vi "LVOBJ to Variant.vi"(8 "error in (no error)":errorcluster, 9 "Variant Type":variant, 10 "JSON Path":string[](array[string]), 11 "Root":T1) -> (0 "error out":errorcluster, 2 "Key":string, 3 "Variant out":variant)   [LabVIEW 2019, in "labview_json.lvlib"]
uses:
  labview_json.lvlib
  Value.ctl
  Value Type.ctl
  <vilib>/Utility/Data Type/Type Definitions/Data Type.ctl
  <vilib>/Utility/error.llb/Error Cluster From Error Code.vi
  <vilib>/ErrorRing/Error Ring.xnode
  <vilib>/Utility/Data Type/NI_Data Type.lvlib
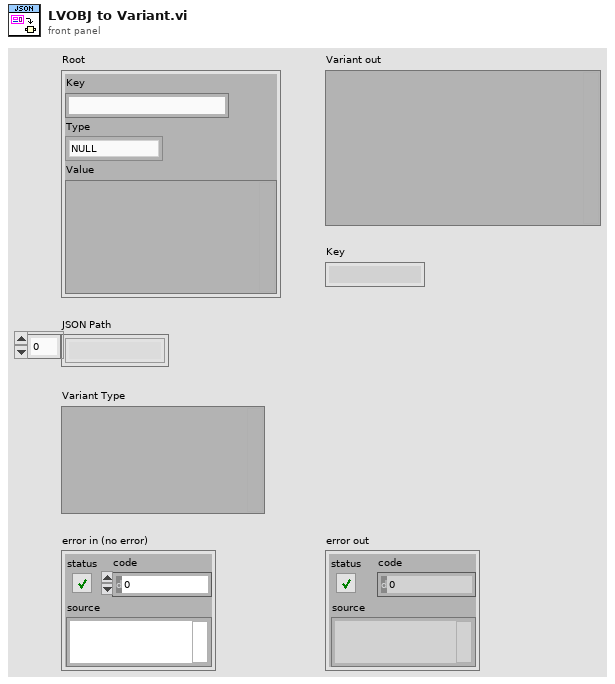
[diagram p1: front panel]
types:
  T1 = typedef "labview_json.lvlib/Value.ctl" = cluster{"Key":string, "Type":T2, "Value":variant}
  T2 = typedef "labview_json.lvlib/Value Type.ctl" = enum8{"NULL", "OBJECT", "ARRAY", "BOOL", "INT", "UINT", "FLOAT", "STRING"}
  T3 = typedef "NI_Data Type.lvlib/Data Type.ctl" = enum8{"Invalid Type", "Void", "I8", "I16", "I32", "I64", "U8", "U16", "U32", "U64", "Single Float", "Double Float", "Extended Float", "Single Complex", "Double Complex", "Extended Complex", "Enum U8", "Enum U16", "Enum U32", "Enum U64", "Single Float With Unit", "Double Float With Unit", "Extended Float With Unit", "Single Complex with Unit", "Double Complex with Unit", "Extended Complex with Unit", "Boolean", "String", "Path", "Picture", "Tag", "Array", "Cluster", "Variant", "LV Variant", "Waveform", "Timestamp", "Digital Waveform", "Digital Data", "ExpressData", "Refnum", "External Data", "VI", "Poly VI", "LabVIEW Class Instance", "Fixed Point", "Set Collection", "Map Collection"}
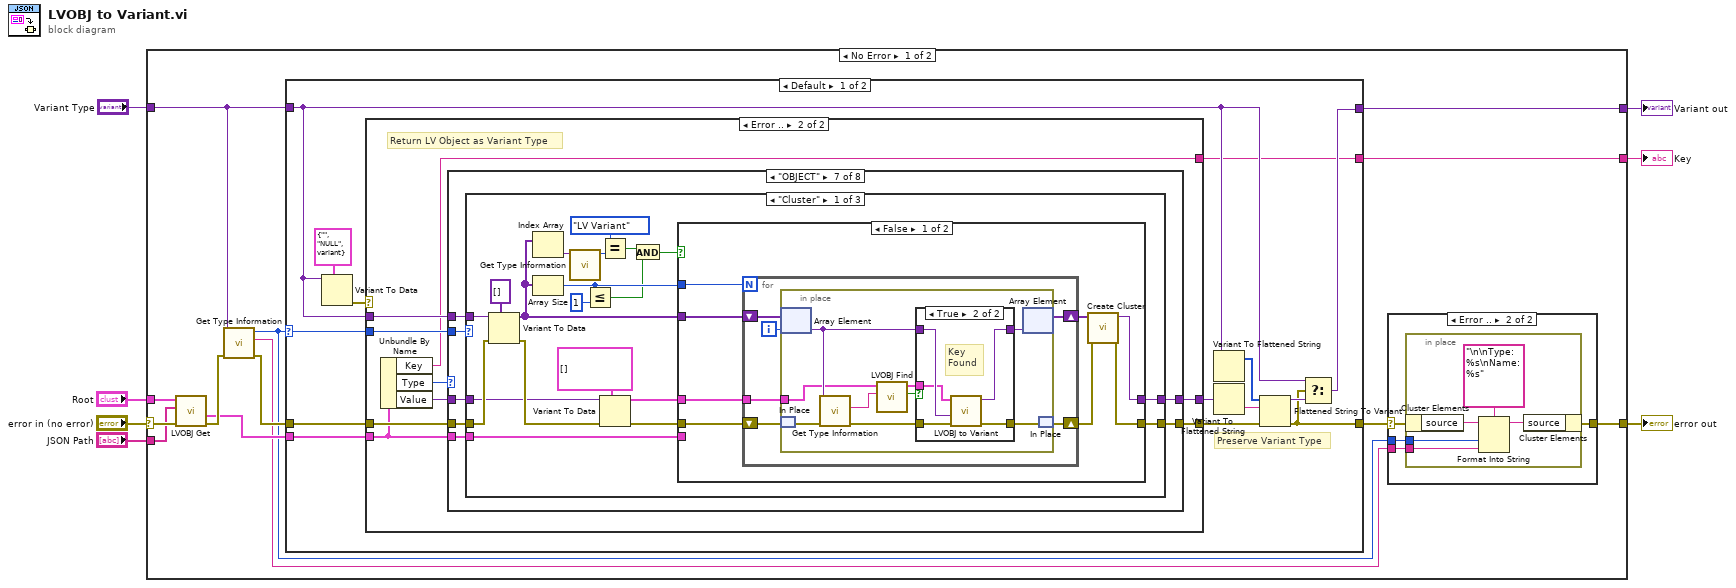
[diagram p0: block diagram]
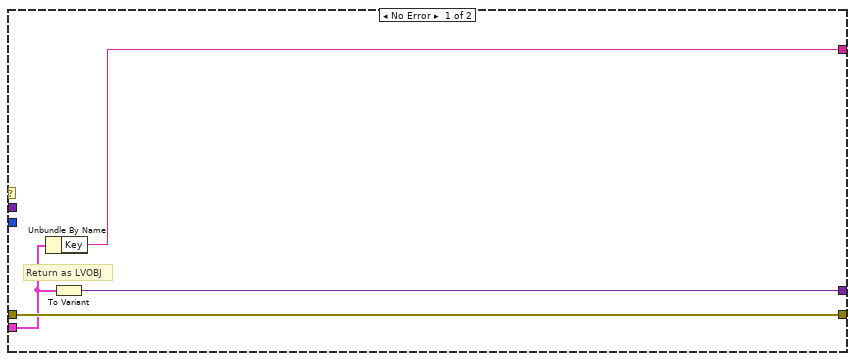
[diagram p3: hidden frame]
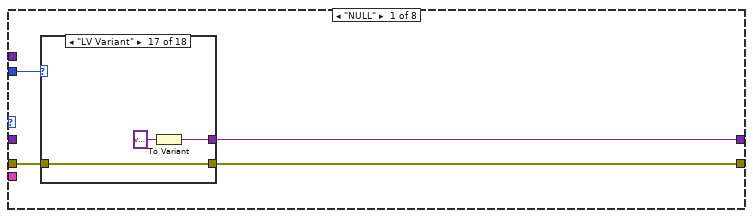
[diagram p4: hidden frame]
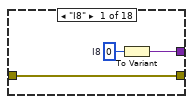
[diagram p5: hidden frame]
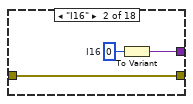
[diagram p6: hidden frame]
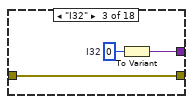
[diagram p7: hidden frame]
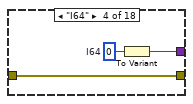
[diagram p8: hidden frame]
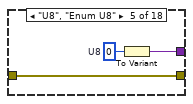
[diagram p9: hidden frame]
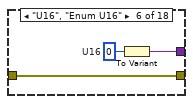
[diagram p10: hidden frame]
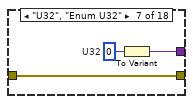
[diagram p11: hidden frame]
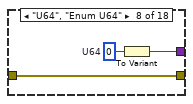
[diagram p12: hidden frame]
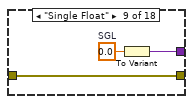
[diagram p13: hidden frame]
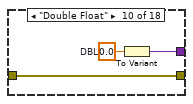
[diagram p14: hidden frame]
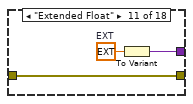
[diagram p15: hidden frame]
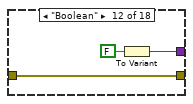
[diagram p16: hidden frame]
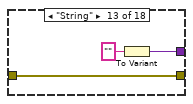
[diagram p17: hidden frame]
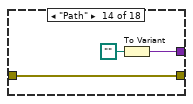
[diagram p18: hidden frame]
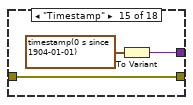
[diagram p19: hidden frame]
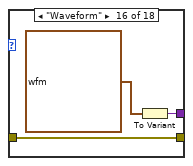
[diagram p20: hidden frame]
diagram:
  n1 = case shown="No Error" "error in (no error)" {
    selector: "error in (no error)" -> [w17 w553]
    tunnel: "Root" -> [w14 _]
    tunnel: [w11 w553] -> w7
    tunnel: [w20 w552] -> w4
    tunnel: "Variant Type" -> [w19 w552]
    tunnel: "JSON Path" -> [w13 _]
    tunnel: [w10 _] -> w1
    frame No Error {
      n2 = call "LVOBJ Get.vi"("error in (no error)"=w17, "JSON Path"=w13, "Element in"=w14) -> ("error out"=w16:errorcluster, "Value"=w15:T1)  [unwired: 5 in, 2 out]
      n3 = call <vilib>:"Get Type Information.vi"("error in (no error)"=w16, "variant"=w19) -> ("error out"=w18:errorcluster, "name"=w8:string, "type"=w9:T3)  [unwired: 5 in, 2 out]
      n4 = case shown="Default" w9 {
        selector: w9 -> [w36 _]
        tunnel: w15 -> [w35 w505]
        tunnel: [w41 w504] -> w12
        tunnel: [w40 w503] -> w20
        tunnel: w18 -> [w38 w500]
        tunnel: w19 -> [w33 _]
        tunnel: [w31 w499] -> w10
        frame Default {
          # "Preserve Variant Type"
          n5 = Variant To Data(type=T1 {"Key"="", "Type"=enum."NULL", "Value"=variant} ("Value"), Variant=w33) -> (error out=w32:errorcluster)  [unwired: 1 in, 1 out]
          n6 = case shown="Error .." w32 {
            tunnel: [w47 w57] -> w39
            tunnel: w38 -> [w47 w56]
            tunnel: [w48 w55] -> w37
            tunnel: w36 -> [_ w54]
            tunnel: w35 -> [w46 w52]
            tunnel: w33 -> [_ w53]
            tunnel: [w45 w49] -> w31
            frame No Error {
              # "Return as LVOBJ"
              n7 = Unbundle By Name(w46) -> ("Key"=w45:string)
              n8 = To Variant(anything=w46) -> (Variant=w48:variant)
            }
            frame Error {
              # "Return LV Object as Variant Type"
              n9 = Unbundle By Name(w52) -> ("Key"=w49:string, "Type"=w51:T2, "Value"=w50:variant)
              n10 = case shown="\"OBJECT\"" w51 {
                tunnel: w56 -> [w58 w123 w134 w193 w252 w312 w366 w461]
                tunnel: [w61 w121 w131 w190 w249 w310 w370 w458] -> w57
                tunnel: w50 -> [_ w122 w133 w192 w251 w311 w364 w460]
                tunnel: w54 -> [w60 w118 w129 w188 w247 w308 w368 w462]
                tunnel: [w59 w117 w128 w187 w246 w307 w365 w456] -> w55
                tunnel: w53 -> [_ _ _ _ _ w304 w369 w459]
                tunnel: w52 -> [_ _ _ _ _ _ w367 w457]
                frame "NULL" {
                  n11 = case shown="\"LV Variant\"" w60 {
                    tunnel: [w64 w67 w70 w73 w76 w79 w82 w85 w88 w91 w94 w97 w100 w103 w106 w109 w112 w115] -> w61
                    tunnel: w58 -> [w64 w67 w70 w73 w76 w79 w82 w85 w88 w91 w94 w97 w100 w103 w106 w109 w112 w115]
                    tunnel: [w63 w66 w69 w72 w75 w78 w81 w84 w87 w90 w93 w96 w99 w102 w105 w108 w111 w114] -> w59
                    frame "I8" {
                      w62 = i8 0  # I8
                      n12 = To Variant(anything=w62) -> (Variant=w63:variant)
                    }
                    frame "I16" {
                      w65 = i16 0  # I16
                      n13 = To Variant(anything=w65) -> (Variant=w66:variant)
                    }
                    frame "I32" {
                      w68 = 0  # I32
                      n14 = To Variant(anything=w68) -> (Variant=w69:variant)
                    }
                    frame "I64" {
                      w71 = i64 0  # I64
                      n15 = To Variant(anything=w71) -> (Variant=w72:variant)
                    }
                    frame "U8", "Enum U8" {
                      w74 = u8 0  # U8
                      n16 = To Variant(anything=w74) -> (Variant=w75:variant)
                    }
                    frame "U16", "Enum U16" {
                      w77 = u16 0  # U16
                      n17 = To Variant(anything=w77) -> (Variant=w78:variant)
                    }
                    frame "U32", "Enum U32" {
                      w80 = u32 0  # U32
                      n18 = To Variant(anything=w80) -> (Variant=w81:variant)
                    }
                    frame "U64", "Enum U64" {
                      w83 = u64 0  # U64
                      n19 = To Variant(anything=w83) -> (Variant=w84:variant)
                    }
                    frame "Single Float" {
                      w86 = sgl 0.0  # SGL
                      n20 = To Variant(anything=w86) -> (Variant=w87:variant)
                    }
                    frame "Double Float" {
                      w89 = 0.0  # DBL
                      n21 = To Variant(anything=w89) -> (Variant=w90:variant)
                    }
                    frame "Extended Float" {
                      w92 = ext 0.0  # EXT
                      n22 = To Variant(anything=w92) -> (Variant=w93:variant)
                    }
                    frame "Boolean" {
                      n23 = To Variant(anything=FALSE) -> (Variant=w96:variant)
                    }
                    frame "String" {
                      n24 = To Variant(anything="") -> (Variant=w99:variant)
                    }
                    frame "Path" {
                      n25 = To Variant(anything=path "" ("Not A Path Constant")) -> (Variant=w102:variant)
                    }
                    frame "Timestamp" {
                      n26 = To Variant(anything=timestamp(0 s since 1904-01-01)) -> (Variant=w105:variant)
                    }
                    frame "Waveform" {
                      n27 = To Variant(anything=waveform(dbl) {"t0"=timestamp(0 s since 1904-01-01), "dt"=1.0, "Y"=[]} ("Waveform")) -> (Variant=w108:variant)
                    }
                    frame "LV Variant" {
                      n28 = To Variant(anything=variant) -> (Variant=w111:variant)
                    }
                    frame Default {
                      n29 = To Variant(anything=variant) -> (Variant=w114:variant)
                    }
                  }
                }
                frame "BOOL" {
                  n30 = Variant To Data(error in=w123, type=FALSE, Variant=w122) -> (data=w120:bool, error out=w121:errorcluster)
                  n31 = To Variant(anything=w120) -> (Variant=w116:variant)
                  n32 = case shown="\"LV Variant\"" w118 {
                    tunnel: [w124 w126] -> w117
                    tunnel: w116 -> [w125 w126]
                    frame "LV Variant" {
                      n33 = To Variant(anything=w125) -> (Variant=w124:variant)
                    }
                    frame Default {
                    }
                  }
                }
                frame "INT" {
                  w132 = i64 0  # I64
                  n34 = Variant To Data(error in=w134, type=w132, Variant=w133) -> (data=w127:i64, error out=w130:errorcluster)
                  n35 = case shown="\"LV Variant\"" w129 {
                    tunnel: [w137 w141 w145 w149 w153 w157 w161 w165 w169 w173 w177 w182 w185] -> w131
                    tunnel: w130 -> [w137 w141 w145 w149 w153 w157 w161 w165 w169 w173 w177 w182 w185]
                    tunnel: [w135 w139 w143 w147 w151 w155 w159 w163 w167 w171 w175 w179 w183] -> w128
                    tunnel: w127 -> [w138 w142 w146 w150 w154 w158 w162 w166 w170 w174 w178 w180 w184]
                    frame "I8" {
                      n36 = To Byte Integer(number=w138) -> (8bit integer=w136:i8)
                      n37 = To Variant(anything=w136) -> (Variant=w135:variant)
                    }
                    frame "I16" {
                      n38 = To Word Integer(number=w142) -> (16bit integer=w140:i16)
                      n39 = To Variant(anything=w140) -> (Variant=w139:variant)
                    }
                    frame "I32" {
                      n40 = To Long Integer(number=w146) -> (32bit integer=w144:i32)
                      n41 = To Variant(anything=w144) -> (Variant=w143:variant)
                    }
                    frame "I64" {
                      n42 = To Quad Integer(1:w150) -> (0:w148:i64)
                      n43 = To Variant(anything=w148) -> (Variant=w147:variant)
                    }
                    frame "U8", "Enum U8" {
                      n44 = To Unsigned Byte Integer(number=w154) -> (unsigned 8bit integer=w152:u8)
                      n45 = To Variant(anything=w152) -> (Variant=w151:variant)
                    }
                    frame "U16", "Enum U16" {
                      n46 = To Unsigned Word Integer(number=w158) -> (unsigned 16bit integer=w156:u16)
                      n47 = To Variant(anything=w156) -> (Variant=w155:variant)
                    }
                    frame "U32", "Enum U32" {
                      n48 = To Unsigned Long Integer(number=w162) -> (unsigned 32bit integer=w160:u32)
                      n49 = To Variant(anything=w160) -> (Variant=w159:variant)
                    }
                    frame "U64", "Enum U64" {
                      n50 = To Unsigned Quad Integer(1:w166) -> (0:w164:u64)
                      n51 = To Variant(anything=w164) -> (Variant=w163:variant)
                    }
                    frame "Single Float" {
                      n52 = To Single Precision Float(number=w170) -> (single precision float=w168:sgl)
                      n53 = To Variant(anything=w168) -> (Variant=w167:variant)
                    }
                    frame "Double Float" {
                      n54 = To Double Precision Float(number=w174) -> (double precision float=w172:dbl)
                      n55 = To Variant(anything=w172) -> (Variant=w171:variant)
                    }
                    frame "Extended Float" {
                      n56 = To Extended Precision Float(1:w178) -> (0:w176:ext)
                      n57 = To Variant(anything=w176) -> (Variant=w175:variant)
                    }
                    frame "LV Variant" {
                      n58 = To Variant(anything=w180) -> (Variant=w181:variant)
                      n59 = To Variant(anything=w181) -> (Variant=w179:variant)
                    }
                    frame Default {
                      n60 = To Variant(anything=w184) -> (Variant=w183:variant)
                    }
                  }
                }
                frame "UINT" {
                  w191 = u64 0  # U64
                  n61 = Variant To Data(error in=w193, type=w191, Variant=w192) -> (data=w186:u64, error out=w189:errorcluster)
                  n62 = case shown="\"LV Variant\"" w188 {
                    tunnel: [w196 w200 w204 w208 w212 w216 w220 w224 w228 w232 w236 w241 w244] -> w190
                    tunnel: w189 -> [w196 w200 w204 w208 w212 w216 w220 w224 w228 w232 w236 w241 w244]
                    tunnel: [w194 w198 w202 w206 w210 w214 w218 w222 w226 w230 w234 w238 w242] -> w187
                    tunnel: w186 -> [w197 w201 w205 w209 w213 w217 w221 w225 w229 w233 w237 w239 w243]
                    frame "I8" {
                      n63 = To Byte Integer(number=w197) -> (8bit integer=w195:i8)
                      n64 = To Variant(anything=w195) -> (Variant=w194:variant)
                    }
                    frame "I16" {
                      n65 = To Word Integer(number=w201) -> (16bit integer=w199:i16)
                      n66 = To Variant(anything=w199) -> (Variant=w198:variant)
                    }
                    frame "I32" {
                      n67 = To Long Integer(number=w205) -> (32bit integer=w203:i32)
                      n68 = To Variant(anything=w203) -> (Variant=w202:variant)
                    }
                    frame "I64" {
                      n69 = To Quad Integer(1:w209) -> (0:w207:i64)
                      n70 = To Variant(anything=w207) -> (Variant=w206:variant)
                    }
                    frame "U8", "Enum U8" {
                      n71 = To Unsigned Byte Integer(number=w213) -> (unsigned 8bit integer=w211:u8)
                      n72 = To Variant(anything=w211) -> (Variant=w210:variant)
                    }
                    frame "U16", "Enum U16" {
                      n73 = To Unsigned Word Integer(number=w217) -> (unsigned 16bit integer=w215:u16)
                      n74 = To Variant(anything=w215) -> (Variant=w214:variant)
                    }
                    frame "U32", "Enum U32" {
                      n75 = To Unsigned Long Integer(number=w221) -> (unsigned 32bit integer=w219:u32)
                      n76 = To Variant(anything=w219) -> (Variant=w218:variant)
                    }
                    frame "U64", "Enum U64" {
                      n77 = To Unsigned Quad Integer(1:w225) -> (0:w223:u64)
                      n78 = To Variant(anything=w223) -> (Variant=w222:variant)
                    }
                    frame "Single Float" {
                      n79 = To Single Precision Float(number=w229) -> (single precision float=w227:sgl)
                      n80 = To Variant(anything=w227) -> (Variant=w226:variant)
                    }
                    frame "Double Float" {
                      n81 = To Double Precision Float(number=w233) -> (double precision float=w231:dbl)
                      n82 = To Variant(anything=w231) -> (Variant=w230:variant)
                    }
                    frame "Extended Float" {
                      n83 = To Extended Precision Float(1:w237) -> (0:w235:ext)
                      n84 = To Variant(anything=w235) -> (Variant=w234:variant)
                    }
                    frame "LV Variant" {
                      n85 = To Variant(anything=w239) -> (Variant=w240:variant)
                      n86 = To Variant(anything=w240) -> (Variant=w238:variant)
                    }
                    frame Default {
                      n87 = To Variant(anything=w243) -> (Variant=w242:variant)
                    }
                  }
                }
                frame "FLOAT" {
                  w250 = 0.0  # DBL
                  n88 = Variant To Data(error in=w252, type=w250, Variant=w251) -> (data=w245:dbl, error out=w248:errorcluster)
                  n89 = case shown="\"LV Variant\"" w247 {
                    tunnel: [w255 w259 w263 w267 w271 w275 w279 w283 w287 w291 w295 w300 w303] -> w249
                    tunnel: w248 -> [w255 w259 w263 w267 w271 w275 w279 w283 w287 w291 w295 w300 w303]
                    tunnel: [w253 w257 w261 w265 w269 w273 w277 w281 w285 w289 w293 w297 w301] -> w246
                    tunnel: w245 -> [w256 w260 w264 w268 w272 w276 w280 w284 w288 w292 w296 w298 w302]
                    frame "I8" {
                      n90 = To Byte Integer(number=w256) -> (8bit integer=w254:i8)
                      n91 = To Variant(anything=w254) -> (Variant=w253:variant)
                    }
                    frame "I16" {
                      n92 = To Word Integer(number=w260) -> (16bit integer=w258:i16)
                      n93 = To Variant(anything=w258) -> (Variant=w257:variant)
                    }
                    frame "I32" {
                      n94 = To Long Integer(number=w264) -> (32bit integer=w262:i32)
                      n95 = To Variant(anything=w262) -> (Variant=w261:variant)
                    }
                    frame "I64" {
                      n96 = To Quad Integer(1:w268) -> (0:w266:i64)
                      n97 = To Variant(anything=w266) -> (Variant=w265:variant)
                    }
                    frame "U8", "Enum U8" {
                      n98 = To Unsigned Byte Integer(number=w272) -> (unsigned 8bit integer=w270:u8)
                      n99 = To Variant(anything=w270) -> (Variant=w269:variant)
                    }
                    frame "U16", "Enum U16" {
                      n100 = To Unsigned Word Integer(number=w276) -> (unsigned 16bit integer=w274:u16)
                      n101 = To Variant(anything=w274) -> (Variant=w273:variant)
                    }
                    frame "U32", "Enum U32" {
                      n102 = To Unsigned Long Integer(number=w280) -> (unsigned 32bit integer=w278:u32)
                      n103 = To Variant(anything=w278) -> (Variant=w277:variant)
                    }
                    frame "U64", "Enum U64" {
                      n104 = To Unsigned Quad Integer(1:w284) -> (0:w282:u64)
                      n105 = To Variant(anything=w282) -> (Variant=w281:variant)
                    }
                    frame "Single Float" {
                      n106 = To Single Precision Float(number=w288) -> (single precision float=w286:sgl)
                      n107 = To Variant(anything=w286) -> (Variant=w285:variant)
                    }
                    frame "Double Float" {
                      n108 = To Double Precision Float(number=w292) -> (double precision float=w290:dbl)
                      n109 = To Variant(anything=w290) -> (Variant=w289:variant)
                    }
                    frame "Extended Float" {
                      n110 = To Extended Precision Float(1:w296) -> (0:w294:ext)
                      n111 = To Variant(anything=w294) -> (Variant=w293:variant)
                    }
                    frame "LV Variant" {
                      n112 = To Variant(anything=w298) -> (Variant=w299:variant)
                      n113 = To Variant(anything=w299) -> (Variant=w297:variant)
                    }
                    frame Default {
                      n114 = To Variant(anything=w302) -> (Variant=w301:variant)
                    }
                  }
                }
                frame "STRING" {
                  n115 = Variant To Data(error in=w312, type="", Variant=w311) -> (data=w306:string, error out=w309:errorcluster)
                  n116 = case shown="\"LV Variant\"" w308 {
                    tunnel: [w315 w319 w323 w327 w329 w340 w351 w363] -> w310
                    tunnel: w309 -> [w315 w319 w323 w327 w328 w339 w350 w363]
                    tunnel: [w314 w316 w322 w326 w338 w349 w360 w361] -> w307
                    tunnel: w306 -> [w313 w317 w321 w325 w335 w346 w357 w362]
                    tunnel: w304 -> [_ _ _ _ w337 w348 w359 _]
                    frame "String" {
                      n117 = To Variant(anything=w313) -> (Variant=w314:variant)
                    }
                    frame "LV Variant" {
                      n118 = To Variant(anything=w317) -> (Variant=w318:variant)
                      n119 = To Variant(anything=w318) -> (Variant=w316:variant)
                    }
                    frame "Path" {
                      n120 = String To Path(string=w321) -> (path=w320:path)
                      n121 = To Variant(anything=w320) -> (Variant=w322:variant)
                    }
                    frame "Timestamp" {
                      n122 = call "ISO8601 to Timestamp.vi"("ISO 8601 Date Time"=w325) -> ("Local Time Stamp"=w324:timestamp)  [unwired: 10 in]
                      n123 = To Variant(anything=w324) -> (Variant=w326:variant)
                    }
                    frame "Enum U8" {
                      n124 = call <vilib>:"Get Numeric Information.vi"("error in (no error)"=w328, "variant"=w337) -> ("error out"=w329:errorcluster, "enum names"=w334:string[])  [unwired: 6 in, 2 out]
                      n125 = Search 1D Array(1D array=w334, element=w335) -> (index of element=w332:i32)  [unwired: 1 in]
                      n126 = Less Than 0?(x=w332) -> (x < 0?=w333:bool)
                      n127 = Select(t=0, s=w333, f=w332) -> (s? t:f=w330:i32)
                      n128 = To Unsigned Byte Integer(number=w330) -> (unsigned 8bit integer=w336:u8)
                      n129 = To Variant(anything=w336) -> (Variant=w338:variant)
                    }
                    frame "Enum U16" {
                      n130 = call <vilib>:"Get Numeric Information.vi"("error in (no error)"=w339, "variant"=w348) -> ("error out"=w340:errorcluster, "enum names"=w345:string[])  [unwired: 6 in, 2 out]
                      n131 = Search 1D Array(1D array=w345, element=w346) -> (index of element=w343:i32)  [unwired: 1 in]
                      n132 = Less Than 0?(x=w343) -> (x < 0?=w344:bool)
                      n133 = Select(t=0, s=w344, f=w343) -> (s? t:f=w341:i32)
                      n134 = To Unsigned Word Integer(number=w341) -> (unsigned 16bit integer=w347:u16)
                      n135 = To Variant(anything=w347) -> (Variant=w349:variant)
                    }
                    frame "Enum U32" {
                      n136 = call <vilib>:"Get Numeric Information.vi"("error in (no error)"=w350, "variant"=w359) -> ("error out"=w351:errorcluster, "enum names"=w356:string[])  [unwired: 6 in, 2 out]
                      n137 = Search 1D Array(1D array=w356, element=w357) -> (index of element=w354:i32)  [unwired: 1 in]
                      n138 = Less Than 0?(x=w354) -> (x < 0?=w355:bool)
                      n139 = Select(t=0, s=w355, f=w354) -> (s? t:f=w352:i32)
                      n140 = To Unsigned Long Integer(number=w352) -> (unsigned 32bit integer=w358:u32)
                      n141 = To Variant(anything=w358) -> (Variant=w360:variant)
                    }
                    frame Default {
                      n142 = To Variant(anything=w362) -> (Variant=w361:variant)
                    }
                  }
                }
                frame "OBJECT" {
                  n143 = case shown="\"Cluster\"" w368 {
                    tunnel: [w390 w431 w444] -> w370
                    tunnel: w366 -> [w386 w433 w445]
                    tunnel: w369 -> [w388 _ w455]
                    tunnel: w367 -> [w371 w434 w446]
                    tunnel: [w389 w430 w435] -> w365
                    tunnel: w364 -> [w372 _ _]
                    frame "Cluster" {
                      n144 = Variant To Data(error in=w386, type=variant[] [], Variant=w388) -> (data=w385:variant[], error out=w375:errorcluster)
                      n145 = Index Array(array=w385) -> (element=w384:variant)  [unwired: 1 in]
                      n146 = Array Size(array=w385) -> (size(s)=w380:i32)
                      n147 = call <vilib>:"Get Type Information.vi"("variant"=w384) -> ("type"=w383:T3)  [unwired: 6 in, 4 out]
                      n148 = Less Or Equal?(x=w380, y=1) -> (x <= y?=w378:bool)
                      n149 = Equal?(x=Data_Type."LV Variant", y=w383) -> (x = y?=w381:bool)
                      n150 = Variant To Data(error in=w375, type=T1[] [], Variant=w372) -> (data=w373:T1[], error out=w374:errorcluster)
                      n151 = And(x=w381, y=w378) -> (x .and. y?=w377:bool)
                      n152 = case shown="False" w377 {
                        tunnel: [w398 w425] -> w390
                        tunnel: [w397 w423] -> w389
                        tunnel: w373 -> [w392 _]
                        tunnel: w374 -> [w391 w428]
                        tunnel: w385 -> [w394 _]
                        tunnel: w380 -> [w393 _]
                        tunnel: w371 -> [_ w421]
                        frame False {
                          n153 = for {
                            N: w393 -> [_]
                            shift-right: [w399] -> w395
                            shift-left: w391 -> [w400]
                            shift-right: [w402] -> w396
                            shift-left: w394 -> [w404]
                            tunnel: w392 -> [w401]
                            i -> [w403]
                            n154 = in-place {
                              in-place-border: w401 -> [w410]
                              n155 = in-place-array #1(w404, w403) -> (w413:variant)
                              n156 = in-place-match #2(w400) -> (w409:errorcluster)
                              n157 = call <vilib>:"Get Type Information.vi"("error in (no error)"=w409, "variant"=w413) -> ("error out"=w408:errorcluster, "name"=w406:string)  [unwired: 5 in, 3 out]
                              n158 = call "LVOBJ Find.vi"("Key"=w406, "Values"=w410) -> ("Found?"=w405:bool, "Value"=w407:T1)  [unwired: 8 in]
                              n159 = case shown="True" w405 {
                                tunnel: w413 -> [w415 w420]
                                tunnel: [w415 w419] -> w412
                                tunnel: [w414 w418] -> w411
                                tunnel: w408 -> [w414 w417]
                                tunnel: w407 -> [_ w416]
                                frame False {
                                # "Key not\nfound,\nreturn type"
                                }
                                frame True {
                                # "Key\nFound"
                                n160 = call "LVOBJ to Variant.vi"("error in (no error)"=w417, "Variant Type"=w420, "Root"=w416) -> ("error out"=w418:errorcluster, "Variant out"=w419:variant)  [unwired: 6 in, 1 out]
                                }
                              }
                              n161 = in-place-array #1(w412) -> (w402:variant[])  [unwired: 1 out]
                              n162 = in-place-match #2(w411) -> (w399:errorcluster)
                            }
                          }
                          n163 = call "Create Cluster.vi"("error in (no error)"=w395, "Elements"=w396) -> ("error out"=w398:errorcluster, "Cluster"=w397:variant)  [unwired: 8 in]
                        }
                        frame True {
                          n164 = call "LVOBJ to Variant.vi"("error in (no error)"=w428, "Variant Type"=variant, "Root"=w421) -> ("error out"=w426:errorcluster, "Variant out"=w427:variant)  [unwired: 6 in, 1 out]
                          n165 = To Variant(anything=w427) -> (Variant=w422:variant)
                          n166 = Build Array(w422) -> (w424:variant[])
                          n167 = call "Create Cluster.vi"("error in (no error)"=w426, "Elements"=w424) -> ("error out"=w425:errorcluster, "Cluster"=w423:variant)  [unwired: 8 in]
                        }
                      }
                    }
                    frame "LV Variant", Default {
                      # "Return as native LV Variant"
                      n168 = call "LVOBJ to Variant.vi"("error in (no error)"=w433, "Variant Type"=variant, "Root"=w434) -> ("error out"=w431:errorcluster, "Variant out"=w430:variant)  [unwired: 6 in, 1 out]
                    }
                    frame "Waveform" {
                      n169 = Variant To Data(error in=w445, type=waveform(dbl) {"t0"=timestamp(0 s since 1904-01-01), "dt"=1.0, "Y"=[]} ("Waveform"), Variant=w455) -> (data=w441:waveform(dbl), error out=w449:errorcluster)
                      n170 = Unbundle By Name(w441) -> ("t0"=w453:timestamp, "dt"=w452:dbl, "Y"=w451:dbl[])
                      n171 = Bundle By Name(cluster=cluster{"t0":timestamp, "dt":dbl, "Y":dbl[]} {"t0"=timestamp(0 s since 1904-01-01), "dt"=0.0, "Y"=[]} ("Waveform"), "t0"=w453, "dt"=w452, "Y"=w451) -> (w442:cluster{"t0":timestamp, "dt":dbl, "Y":dbl[]})
                      n172 = To Variant(anything=w442) -> (Variant=w447:variant)
                      n173 = call "LVOBJ to Variant.vi"("error in (no error)"=w449, "Variant Type"=w447, "Root"=w446) -> ("error out"=w448:errorcluster, "Variant out"=w443:variant)  [unwired: 6 in, 1 out]
                      n174 = Variant To Data(error in=w448, type=w442, Variant=w443) -> (data=w440:cluster{"t0":timestamp, "dt":dbl, "Y":dbl[]}, error out=w444:errorcluster)
                      n175 = Unbundle By Name(w440) -> ("t0"=w437:timestamp, "dt"=w438:dbl, "Y"=w439:dbl[])
                      n176 = Bundle By Name(cluster=w441, "t0"=w437, "dt"=w438, "Y"=w439) -> (w436:waveform(dbl))
                      n177 = To Variant(anything=w436) -> (Variant=w435:variant)
                    }
                  }
                }
                frame "ARRAY" {
                  n178 = case shown="\"Array\"" w462 {
                    tunnel: w461 -> [w472 w497]
                    tunnel: w460 -> [w471 _]
                    tunnel: w459 -> [w465 _]
                    tunnel: [w467 w495] -> w458
                    tunnel: w457 -> [_ w496]
                    tunnel: [w464 w494] -> w456
                    frame "Array" {
                      n179 = Variant To Data(error in=w472, type=T1[] [], Variant=w471) -> (data=w466:T1[], error out=w470:errorcluster)
                      n180 = call <vilib>:"Get Array Information.vi"("error in (no error)"=w470, "variant"=w465) -> ("error out"=w468:errorcluster, "array element data type"=w463:variant, "number of dimensions"=w469:i32)  [unwired: 6 in, 1 out]
                      n181 = case shown="1" w469 {
                        tunnel: w468 -> [w479 w489]
                        tunnel: [w477 w488] -> w467
                        tunnel: w466 -> [w480 _]
                        tunnel: w465 -> [_ w486]
                        tunnel: [w474 w486] -> w464
                        tunnel: w463 -> [w475 _]
                        frame 1 {
                          n182 = for {
                            tunnel: w480 -> [w481] mode=indexing
                            shift-right: [w484] -> w478
                            shift-left: w479 -> [w485]
                            tunnel: w475 -> [w483]
                            tunnel: [w482] -> w476 mode=indexing
                            n183 = call "LVOBJ to Variant.vi"("error in (no error)"=w485, "Variant Type"=w483, "Root"=w481) -> ("error out"=w484:errorcluster, "Variant out"=w482:variant)  [unwired: 6 in, 1 out]
                          }
                          n184 = call "Create Array.vi"("error in (no error)"=w478, "Default Type (if empty)"=w475, "Elements"=w476) -> ("error out"=w477:errorcluster, "Array"=w474:variant)  [unwired: 7 in]
                        }
                        frame Default {
                          n185 = xnode "Error Ring"() -> ("error out"=w487:errorcluster)
                          n186 = Merge Errors(w489, w487) -> (w488:errorcluster)
                        }
                      }
                    }
                    frame "LV Variant", Default {
                      # "Return as native LV Variant"
                      n187 = call "LVOBJ to Variant.vi"("error in (no error)"=w497, "Variant Type"=variant, "Root"=w496) -> ("error out"=w495:errorcluster, "Variant out"=w494:variant)  [unwired: 6 in, 1 out]
                    }
                  }
                }
              }
            }
          }
          n188 = Variant To Flattened String(Variant=w33) -> (1:w42:i16[])  [unwired: 1 out]
          n189 = Variant To Flattened String(Variant=w37) -> (data string=w44:string)  [unwired: 1 out]
          n190 = Flattened String To Variant(4:w39, 6:w44, 7:w42) -> (0:w41:errorcluster, 3:w43:variant)
          n191 = Select(t=w33, s=w41, f=w43) -> (s? t:f=w40:variant)
        }
        frame "Void" {
          # "Return native LV object as a variant"
          n192 = Unbundle By Name(w505) -> ("Key"=w499:string, "Type"=w502:T2, "Value"=w501:variant)
          n193 = case shown="\"ARRAY\"" w502 {
            tunnel: w501 -> [_ w520 w542 w551]
            tunnel: w499 -> [_ _ _ _]
            tunnel: w500 -> [w508 w518 w540 w550]
            tunnel: [w508 w511 w538 w550] -> w504
            tunnel: [w506 w509 w535 w551] -> w503
            frame "NULL" {
              # "Empty Variant"
              n194 = To Variant(anything=variant ("variant")) -> (Variant=w506:variant)
            }
            frame "OBJECT" {
              n195 = Variant To Data(error in=w518, type=T1[] [], Variant=w520) -> (data=w516:T1[], error out=w517:errorcluster)
              n196 = for {
                tunnel: w516 -> [w533] mode=indexing
                shift-right: [w531] -> w514
                shift-left: w517 -> [w534]
                tunnel: [w532] -> w515 mode=indexing
                tunnel: [w530] -> w513 mode=indexing
                n197 = call "LVOBJ to Variant.vi"("error in (no error)"=w534, "Root"=w533) -> ("error out"=w531:errorcluster, "Key"=w530:string, "Variant out"=w532:variant)  [unwired: 7 in]
              }
              n198 = for {
                tunnel: w515 -> [w527] mode=indexing
                tunnel: w513 -> [w528] mode=indexing
                shift-right: [w523] -> w512
                shift-left: w514 -> [w529]
                tunnel: [w521] -> w510 mode=indexing
                n199 = call <vilib>:"Set Type Information.vi"("error in (no error)"=w529, "Name"=w528, "Variant in"=w527) -> ("error out"=w524:errorcluster, "Variant out"=w526:variant)  [unwired: 7 in]
                n200 = Variant To Flattened String(Variant=w527) -> (data string=w522:string)  [unwired: 1 out]
                n201 = Variant To Flattened String(Variant=w526) -> (1:w525:i16[])  [unwired: 1 out]
                n202 = Flattened String To Variant(4:w524, 6:w522, 7:w525) -> (0:w523:errorcluster, 3:w521:variant)
              }
              n203 = call "Create Cluster.vi"("error in (no error)"=w512, "Elements"=w510) -> ("error out"=w511:errorcluster, "Cluster"=w509:variant)  [unwired: 8 in]
            }
            frame "ARRAY" {
              n204 = Variant To Data(error in=w540, type=T1[] [], Variant=w542) -> (data=w537:T1[], error out=w539:errorcluster)
              n205 = for {
                tunnel: w537 -> [w549] mode=indexing
                shift-right: [w546] -> w538
                shift-left: w539 -> [w548]
                tunnel: [w543] -> w536 mode=indexing
                n206 = call "LVOBJ to Variant.vi"("error in (no error)"=w548, "Root"=w549) -> ("error out"=w547:errorcluster, "Variant out"=w545:variant)  [unwired: 7 in, 1 out]
                n207 = Variant To Data(error in=w547, type=variant, Variant=w545) -> (data=w543:variant, error out=w546:errorcluster)
              }
              n208 = To Variant(anything=w536) -> (Variant=w535:variant)
            }
            frame "BOOL".."STRING" {
            }
          }
        }
      }
      n209 = case shown="Error .." w12 {
        selector: w12 -> [w21 w25]
        tunnel: [w21 w24] -> w11
        tunnel: w9 -> [_ w23]
        tunnel: w8 -> [_ w22]
        frame No Error {
        }
        frame Error {
          n210 = in-place {
            in-place-border: w23 -> [w27]
            in-place-border: w22 -> [w26]
            n211 = in-place-cluster #3(w25) -> ("source"=w30:string)
            n212 = Format Into String(format string="\n\nType: %s\nName: %s", initial string=w30, w27, w26) -> (resulting string=w29:string)  [unwired: 1 in, 1 out]
            n213 = in-place-cluster #3("source"=w29) -> (w24:errorcluster)
          }
        }
      }
    }
    frame Error {
    }
  }
  "error out" <- w7
  "Variant out" <- w4
  "Key" <- w1
